vi "Edytuj_TDMS_laucher.vi"() -> ()   [LabVIEW 2013]
doc: "Use this template to build a standard state machine design pattern. Each state executes code and determines which state to transition to. Contrast this design pattern with the User Interface Event Handler pattern, in which code executes in response to user actions. Contrast this design pattern also with the Queued Message Handler pattern, in which each message handling code can queue zero or more new messages.\nNote: This template does not contain the most recent programming guidelines recommended by National Instruments. For a complete, project-based implementation of the Standard State Machine pattern, use the Create Project dialog box instead of this template."
uses:
  Kontrolki/TDMS_read/TDMS__czytaj_stany.ctl
panel:
  out "Podglad":waveform(dbl)[](graph)
  in  "Rezygnuj":bool
  in  "Edytuj":bool
  in  "Lista pomiarów":i32(listbox)
  out "Stan":T1
  in  "Wczytaj":bool
  in  "Podglad":bool
  in  "Wczytaj plik TDMS":path
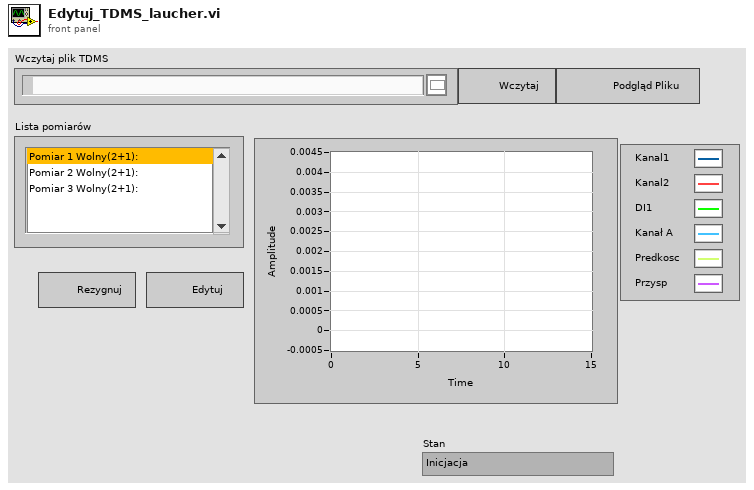
[diagram p1: front panel]
types:
  T1 = typedef "TDMS__czytaj_stany.ctl" = enum16{"Inicjacja", "Wczytaj_Plik", "Podglad", "L_Grup", "Wybierz_grupe", "Wyswietl_grupe", "Zatwierdz", "Error"}
  T2 = typedef "Kanaly.ctl" = cluster{"Analogowe":waveform(dbl)[], "Cyfrowe":waveform(dbl)[], "Zwarcie":waveform(dbl)[], "Enkoder":waveform(dbl)[]}
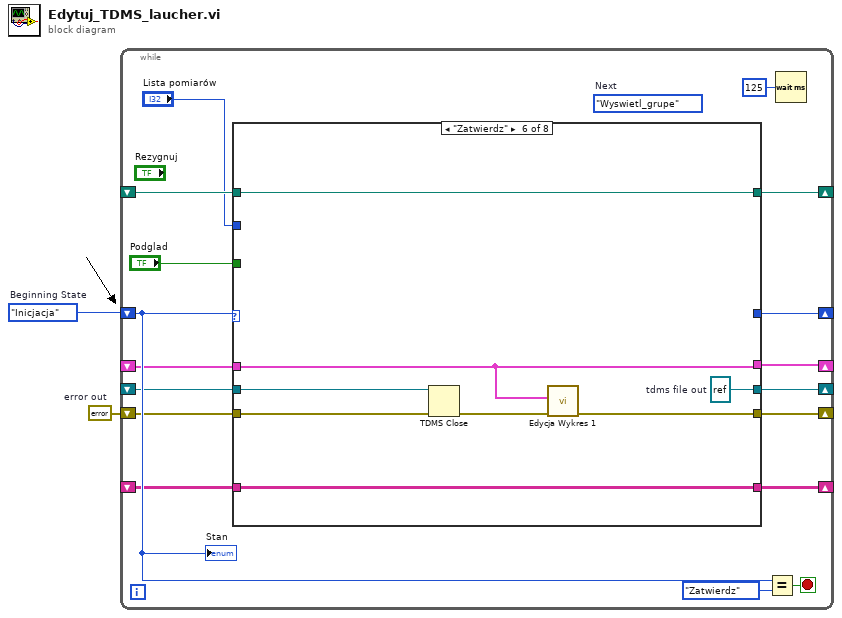
[diagram p0: block diagram]
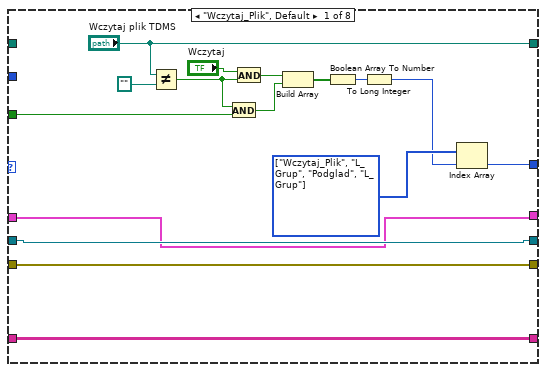
[diagram p2: hidden frame]
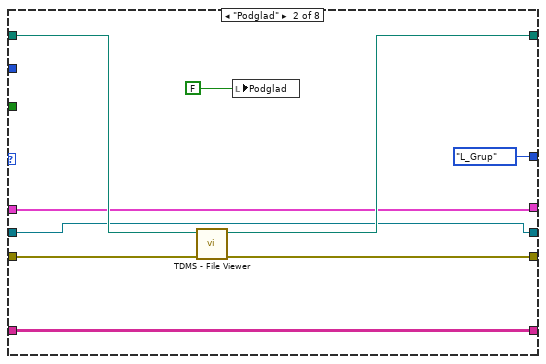
[diagram p3: hidden frame]
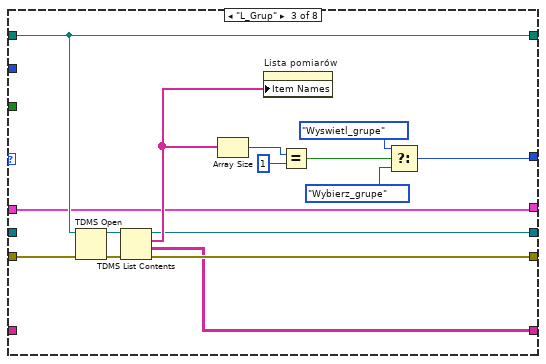
[diagram p4: hidden frame]
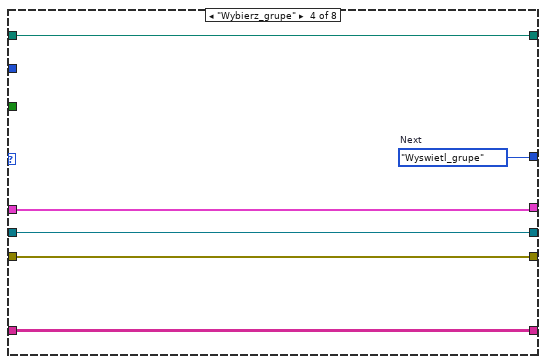
[diagram p5: hidden frame]
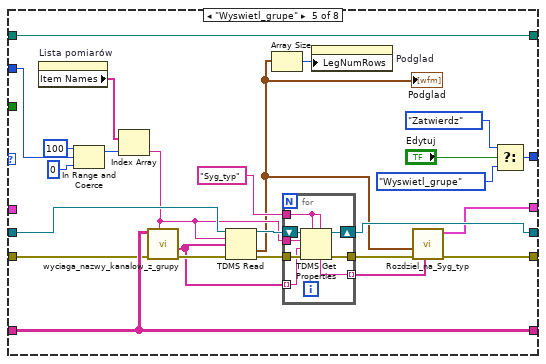
[diagram p6: hidden frame]
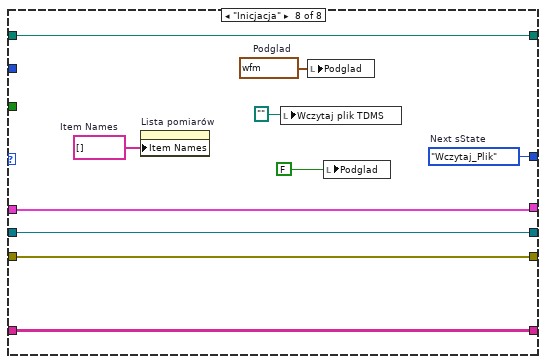
[diagram p8: hidden frame]
diagram:
  w1 = errorcluster {"status"=FALSE, "code"=0, "source"=""}  # error out
  w2 = TDMS__czytaj_stany."Inicjacja"  # Beginning State
  n1 = while {
    shift-right: [w16] -> _
    shift-left: w2 -> [w17]
    shift-right: [w14] -> _
    shift-left: _ -> [w12]
    shift-right: [w10] -> _
    shift-left: w1 -> [w11]
    shift-right: [w9] -> _
    shift-left: _ -> [w8]
    shift-right: [w6] -> _
    shift-left: _ -> [w5]
    shift-right: [w4] -> _
    shift-left: _ -> [w3]
    stop <- w19 stop-if-true
    (unwired) TDMS__czytaj_stany."Wyswietl_grupe"  # Next
    n2 = case shown="\"Zatwierdz\"" w17 {
      tunnel: [w31 TDMS__czytaj_stany."L_Grup" ("Next State") w51 w61 w82 _ _ w120] -> w16
      tunnel: ["Wczytaj plik TDMS" w42 w58 w65 w91 w107 w112 w119] -> w14
      tunnel: "Podglad" -> [w23 _ _ _ _ _ _ _]
      tunnel: w12 -> [_ w43 w58 w65 w91 w107 w112 w119]
      tunnel: w11 -> [w28 w41 w49 w64 w87 w106 w111 w118]
      tunnel: [w28 w40 w48 w64 w70 w101 w111 w118] -> w10
      tunnel: [w22 w38 w47 w63 w79 w104 w110 w116] -> w9
      tunnel: w8 -> [w22 w38 _ w63 w88 w105 w110 w116]
      tunnel: "Lista pomiarów" -> [_ _ _ _ w75 _ _ _]
      tunnel: [w21 w37 w46 w62 w90 w103 w109 w115] -> w6
      tunnel: w5 -> [w21 w37 _ w62 w90 w103 w109 w115]
      tunnel: [w20 w36 w45 w60 w69 w100 w108 w114] -> w4
      tunnel: w3 -> [w20 w36 w45 w60 _ w100 w108 w114]
      frame "Wczytaj_Plik", Default {
        w32 = T1[] [enum."Wczytaj_Plik", enum."L_Grup", enum."Podglad", enum."L_Grup"] items=["Inicjacja", "Wczytaj_Plik", "Podglad", "L_Grup", "Wybierz_grupe", "Wyswietl_grupe", "Zatwierdz", "Error"]
        n3 = Not Equal?(x="Wczytaj plik TDMS", y=path "") -> (x != y?=w24:bool)
        n4 = And(x=w24, y=w23) -> (x .and. y?=w25:bool)
        n5 = And(x="Wczytaj", y=w24) -> (x .and. y?=w26:bool)
        n6 = Build Array(w26, w25) -> (w33:bool[])
        n7 = Boolean Array To Number(Boolean array=w33) -> (number=w30:u32)
        n8 = To Long Integer(number=w30) -> (32bit integer=w29:i32)
        n9 = Index Array(array=w32, index=w29) -> (element=w31:T1)
      }
      frame "Podglad" {
        n10 = call <vilib>:"TDMS - File Viewer.vi"("error in (no error)"=w41, "file path"=w43) -> ("error out"=w40:errorcluster, "file path out"=w42:path)  [unwired: 4 in]
        n11 = local write "Podglad"(FALSE ("Podglad")) -> ()
      }
      frame "L_Grup" {
        n12 = TDMS Open(8:w49, 11:w58) -> (0:w57:errorcluster, 3:w59:refnum<k34>)  [unwired: 5 in]
        n13 = TDMS List Contents(4:w57, 7:w59) -> (0:w48:errorcluster, 1:w46:string[][], 2:w56:string[], 3:w47:refnum<k34>)  [unwired: 1 in]
        n14 = Array Size(array=w56) -> (size(s)=w55:i32)
        n15 = property on="Lista pomiarów" class="LstBox (strict)"("Item Names"=w56) -> ()  [unwired: 2 in, 2 out]
        n16 = Equal?(x=w55, y=1) -> (x = y?=w53:bool)
        n17 = Select(t=TDMS__czytaj_stany."Wyswietl_grupe" ("Next"), s=w53, f=TDMS__czytaj_stany."Wybierz_grupe" ("Next")) -> (s? t:f=w51:T1)
      }
      frame "Wybierz_grupe" {
        w61 = TDMS__czytaj_stany."Wyswietl_grupe"  # Next
      }
      frame "Wyswietl_grupe" {
        n18 = property on="Lista pomiarów" class="LstBox (strict)"() -> ("Item Names"=w89:string[])  [unwired: 2 in, 2 out]
        n19 = In Range and Coerce(upper limit=100, x=w75, lower limit=0 ("upper limit")) -> (coerced(x)=w72:i32)  [unwired: 1 out]
        n20 = Index Array(array=w89, index=w72) -> (element=w77:string)
        n21 = call "wyciaga_nazwy_kanalow_z_grupy.vi"("Group"=w77, "error in (no error)"=w87, "group/channel names"=w90) -> ("error out"=w86:errorcluster, "channel names"=w76:string[])  [unwired: 7 in]
        n22 = TDMS Read(0:w88, 5:w77, 7:w76, 11:w86) -> (4:w81:refnum<k34>, 10:w66:waveform(dbl)[], 15:w80:errorcluster)  [unwired: 4 in, 3 out]
        "Podglad" <- w66
        n23 = Array Size(array=w66) -> (size(s)=w67:i32)
        n24 = for {
          tunnel: w80 -> [w98]
          tunnel: [w96] -> w71
          tunnel: w77 -> [w95]
          tunnel: w76 -> [w94] mode=indexing
          shift-right: [w97] -> w79
          shift-left: w81 -> [w99]
          tunnel: "Syg_typ" -> [w93]
          tunnel: [w92] -> w68 mode=indexing
          n25 = TDMS Get Properties(5:w93, 7:w93, 8:w98, 9:w94, 10:w95, 11:w99) -> (0:w96:errorcluster, 3:w97:refnum<k34>, 4:w92:string)  [unwired: 3 out]
        }
        n26 = property on="Podglad" class="WFGraph (strict)"("LegNumRows"=w67) -> ()  [unwired: 2 in, 2 out]
        n27 = call "Rozdziel_na_Syg_typ.vi"("Property Syg_typ"=w68, "error in (no error)"=w71, "data"=w66) -> ("error out"=w70:errorcluster, "Przebiegi"=w69:T2)  [unwired: 7 in]
        n28 = Select(t=TDMS__czytaj_stany."Zatwierdz" ("Next"), s="Edytuj", f=TDMS__czytaj_stany."Wyswietl_grupe" ("Next")) -> (s? t:f=w82:T1)
      }
      frame "Zatwierdz" {
        w104 = refnum<k34> refnum  # tdms file out
        n29 = TDMS Close(8:w106, 11:w105) -> (0:w102:errorcluster)  [unwired: 1 out]
        n30 = call "Edycja Wykres 1.vi"("error in (no error)"=w102, "Data in"=w100) -> ("error out"=w101:errorcluster)  [unwired: 9 in]
      }
      frame "Error" {
      }
      frame "Inicjacja" {
        w113 = waveform(dbl)[] [{"t0"=timestamp(0 s since 1904-01-01), "dt"=0.2, "Y"=[3.984629926233525e-06, 3.5996723334995685e-06, -9.103928309739926e-06, 2.4447995463718323e-06, -3.714521979048707e-06, -5.260413656616714e-05, -4.1440366306172206e-05, 1.283865461720381e-05, 2.361746728695981e-05, -1.064375868861798e-05, -5.183422137431681e-05, -2.873676566266868e-05, 3.054670399290602e-05, 6.249818440248248e-05, 2.015284892569714e-05, 1.3993527404043414e-05, 3.093166159506946e-05, 2.708208564220024e-05, 1.476344259111889e-05, 5.248928692438461e-05, -8.71897070999997e-06, -8.334013117026135e-06, 1.1683781835186676e-05, 2.0598419519823536e-06, 1.8228060951422138e-05, 2.900687361793898e-05, 2.8621916020766353e-05, 2.9006873619618554e-05, 2.0152848928480504e-05, 1.8997976141232865e-05, 4.402021983061121e-05, 1.9767891332747233e-05, 4.402021983248244e-05, 1.6303272976043262e-05, 5.9094179019482374e-06, 1.899797614159277e-05, 2.7082085641528597e-05, 4.2095431855304185e-05, 2.4002424876670818e-05, -1.3338461856950691e-05, 1.3223612215648201e-05, 1.9767891333131244e-05, 2.8297571426328473e-06, 6.294375503703919e-06, 2.7082085638721218e-05, 1.0528909045875865e-05, 1.6688230572664054e-05, 1.7458145759307915e-05, -1.025880109310065e-05, -1.0258801092788817e-05, -5.639309951644459e-06, 4.75454511789193e-06, 2.1692679306950292e-05, -1.1028716282887709e-05, -2.49903618050044e-07, -1.0258801094972048e-05, 1.4378485000136401e-05, 9.37403626299487e-06, 1.938293373658228e-05, -9.488885901058456e-06, 1.9382933737205748e-05, 2.7082085638577368e-05, 8.989078667765602e-06, 1.3223612216655913e-05, -1.3338461852632077e-05, 3.599672334387228e-06, 4.05556014763544e-05, 2.207763690208383e-05, 1.5533357783401096e-05, 1.6688230571560417e-05], "attributes"=variant("NI_ChannelName"=variant(string "Kanal1"), "Syg_typ"=variant(string "A"))}, {"t0"=timestamp(0 s since 1904-01-01), "dt"=0.2, "Y"=[0.00430061120196013, 0.004282133237374443, 0.004299071371577175, 0.004306770523486247, 0.0043194741241439, 0.004290987262073831, 0.004281363322180961, 0.004295606753219246, 0.004314469675405295, 0.004294451880427277, 0.004299841286770702, 0.004281748279776313, 0.004343726452669611, 0.004319089166549918, 0.004283673067748815, 0.004322938742507128, 0.004302151032347235, 0.004327173276057554, 0.0042705845095026935, 0.004315239590594604, 0.004327943191248011, 0.004323323700103772, 0.0043437264526688685, 0.00433102285201589, 0.004295991710813396, 0.004308310353873998, 0.0042859828133240034, 0.004300226244368691, 0.0043290980640369615, 0.004306000608297322, 0.0042825181949660025, 0.004314469675405943, 0.004309080269065968, 0.004299456329175809, 0.0043129298450194364, 0.004290602304476636, 0.004302920947533354, 0.004312929845023802, 0.0043086953114730665, 0.004307155481087519, 0.004291757177261078, 0.004304075820320816, 0.0043133148026171355, 0.004333717555187676, 0.004322553784913937, 0.004331407809611288, 0.00433140780961052, 0.004343341495071913, 0.004292912050048827, 0.004316009505784485, 0.004300611201963319, 0.004319474124147331, 0.0043048457355108205, 0.004314469675404097, 0.004306385565893152, 0.0042963766684065655, 0.004308695311471962, 0.004346036198245136, 0.004345266283055443, 0.004306770523490299, 0.004304845735512738, 0.004334487470374489, 0.0043225537849127405, 0.00432024403933611, 0.004334102512780146, 0.004308695311469036, 0.004301381117152413, 0.00429137221966918, 0.004303305905132707, 0.004301381117155147], "attributes"=variant("NI_ChannelName"=variant(string "Kanal2"), "Syg_typ"=variant(string "A"))}, {"t0"=timestamp(3542365949.9265184 s since 1904-01-01), "dt"=0.0003125, "Y"=array[44800 elements], "attributes"=variant("Aktywny"=variant(bool TRUE), "NI_ChannelName"=variant(string "DI1"), "NI_UnitDescription"=variant(string "Volts"), "NO"=variant(i32 0), "Syg_typ"=variant(string "C"), "Typ"=variant(string "DI"))}, {"t0"=timestamp(0 s since 1904-01-01), "dt"=0.5, "Y"=[0.0, 0.0, 0.0, 0.0, 0.0, 0.0, 0.0, 0.0, 0.0, 0.0, 0.0, 0.0, 0.0, 0.0, 0.0, 0.0, 0.0, 0.0, 0.0, 0.0, 0.0, 0.0, 0.0, 0.0, 0.0, 0.0, 0.0, 0.0], "attributes"=variant("NI_ChannelName"=variant(string "Kana³ A"), "Syg_typ"=variant(string "E"), "Typ"=variant(string "EN"))}, {"t0"=timestamp(0 s since 1904-01-01), "dt"=0.5, "Y"=[0.0, 0.0, 0.0, 0.0, 0.0, 0.0, 0.0, 0.0, 0.0, 0.0, 0.0, 0.0, 0.0, 0.0, 0.0, 0.0, 0.0, 0.0, 0.0, 0.0, 0.0, 0.0, 0.0, 0.0, 0.0, 0.0, 0.0, 0.0], "attributes"=variant("NI_ChannelName"=variant(string "Predkosc"), "Syg_typ"=variant(string "E"), "Typ"=variant(string "EN"))}, {"t0"=timestamp(0 s since 1904-01-01), "dt"=0.5, "Y"=[0.0, 0.0, 0.0, 0.0, 0.0, 0.0, 0.0, 0.0, 0.0, 0.0, 0.0, 0.0, 0.0, 0.0, 0.0, 0.0, 0.0, 0.0, 0.0, 0.0, 0.0, 0.0, 0.0, 0.0, 0.0, 0.0, 0.0, 0.0], "attributes"=variant("NI_ChannelName"=variant(string "Przysp"), "Syg_typ"=variant(string "E"), "Typ"=variant(string "EN"))}]  # Podglad
        w117 = string[] []  # Item Names
        w120 = TDMS__czytaj_stany."Wczytaj_Plik"  # Next sState
        n31 = property on="Lista pomiarów" class="LstBox (strict)"("Item Names"=w117) -> ()  [unwired: 2 in, 2 out]
        n32 = local write "Wczytaj plik TDMS"(path "") -> ()
        n33 = local write "Podglad"(w113) -> ()
        n34 = local write "Podglad"(FALSE ("Podglad")) -> ()
      }
    }
    n35 = Equal?(x=w17, y=TDMS__czytaj_stany."Zatwierdz" ("States")) -> (x = y?=w19:bool)
    n36 = Wait (ms)(milliseconds to wait=u32 125) -> ()  [unwired: 1 out]
    "Stan" <- w17
  }
